vi "f_11_DvDtOff.vi"(0 "file path (IN)":path, 1 "Project #":string, 2 "Request #":string, 3 "TEST #":string, 5 "error in (no error)":errorcluster, 6 "VCE":dbl) -> (11 "Dv (V)":dbl, 13 "Dt (ns)":dbl, 14 "file path (OUT)":path, 15 "Dv/Dt (V/us)":dbl, 16 "DONE Dv/Dt OFF":bool, 19 "error out":errorcluster)   [LabVIEW 2020]
uses:
  GlobIndSw1.vi
  <vilib>/Waveform/WDTOps.llb/WDT Waveform Duration DBL.vi
  <vilib>/Waveform/WDTOps.llb/WDT Get Waveform Subset DBL.vi
  <vilib>/measure/mamon.llb/Trigger Detection for 1 Channel.vi
  <vilib>/Analysis/NI_AALBase.lvlib
  <vilib>/measure/NI_MAPro.lvlib
panel:
  in  "Decision ?":bool
  out "Dt (us)":dbl
  out "80% Vce":dbl
  out "50% Vce":dbl
  out "Cursor a : Channel 3":dbl
  out "Cursor b : Channel 3":dbl
  out "Waveform Graph":waveform(dbl)[](graph)
  out "OFF Region":waveform(dbl)[](graph) caption="DvDt off (V/us)"
  # "Dv/dt(off): from 50% to 80% of the peak voltage"
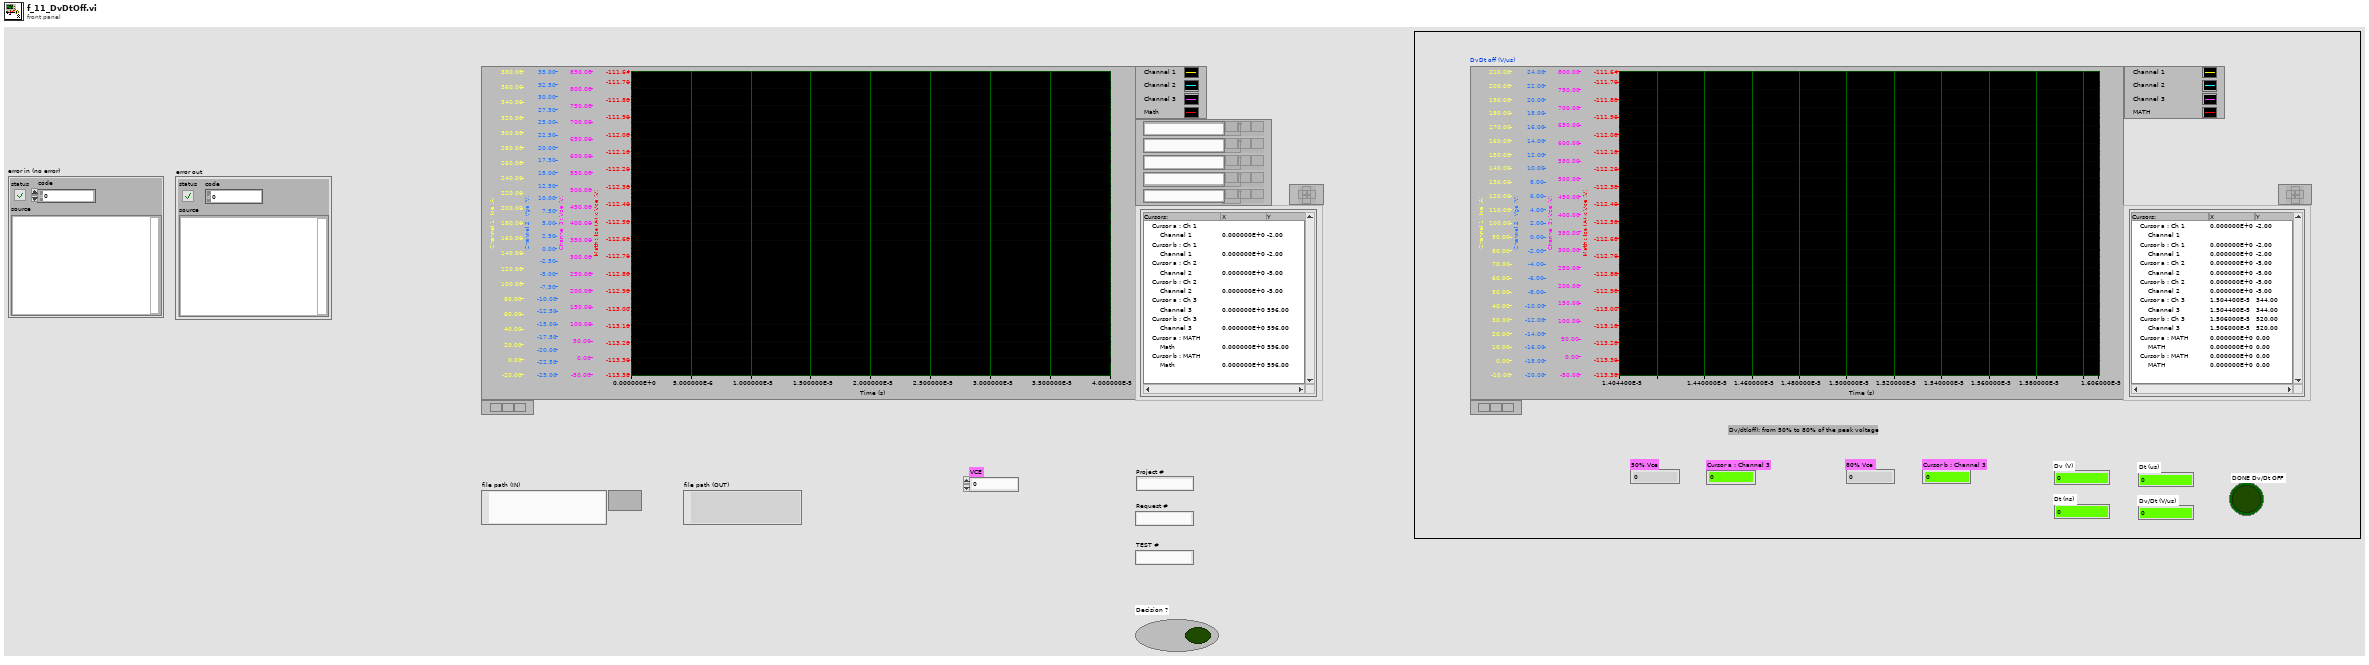
[diagram p1: front panel]
types:
  T1 = enum32{"Invalid", "Standard", "Closed", "Hidden", "Minimized", "Maximized"}
  T2 = typedef "imagedata.ctl" = cluster{"image type":i32, "image depth":i32, "image":u8[], "mask":u8[], "colors":u32[], "Rectangle":cluster{"left":i16, "top":i16, "right":i16, "bottom":i16}}
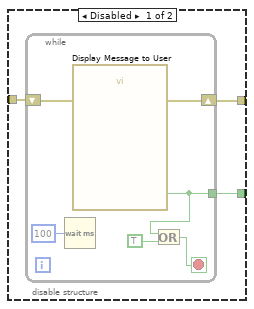
[diagram p2: hidden frame]
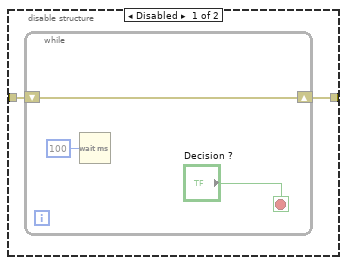
[diagram p7: hidden frame]
diagram:
  w2 = 0.0 ("Dv (V)")
  w3 = errorcluster {"status"=FALSE, "code"=0, "source"=""} ("error out")
  w1 = FALSE ("DONE Tdon")
  w4 = waveform(dbl)[] [] ("Waveform Graph")
  n1 = local write "error out"(w3) -> ()
  n2 = local write "error in (no error)"(w3) -> ()
  n3 = local write "DONE Dv/Dt OFF"(w1) -> ()
  n4 = local write "Waveform Graph"(w4) -> ()
  n5 = local write "OFF Region"(w4) -> ()
  n6 = local write "Decision ?"(w1) -> ()
  n7 = local write "Dv (V)"(w2) -> ()
  n8 = local write "Dt (ns)"(w2) -> ()
  n9 = local write "Dt (us)"(w2) -> ()
  n10 = local write "Dv/Dt (V/us)"(w2) -> ()
  n11 = local write "Cursor a : Channel 3"(w2) -> ()
  n12 = local write "Cursor b : Channel 3"(w2) -> ()
  n13 = flat-sequence {
    tunnel: ["error in (no error)"] -> w10
    tunnel: ["file path (IN)"] -> w9
    tunnel: [w21] -> w8
    tunnel: [w20] -> w7
    tunnel: w10 -> [w19]
    tunnel: w9 -> [w18]
    tunnel: [w279] -> w6
    tunnel: w8 -> [w278]
    tunnel: w7 -> [w277]
    tunnel: [w277] -> w5
    tunnel: w6 -> [w292]
    tunnel: w5 -> [w293]
    frame #0 {
      n14 = control-ref of="This VI"() -> (w15:refnum<vi>)
      n15 = invoke class="VI" method="FP.Open"(reference=w15, error in="error in (no error)", "Activate"=TRUE ("Activate?"), "State"=T1."Maximized") -> (error out=w16:errorcluster)  [unwired: 1 in, 4 out]
      n16 = property class="VI"(reference=w15, error in=w16, "Front Panel.Closeable"=TRUE ("Front Panel Window:Closeable")) -> ()  [unwired: 2 out]
    }
    frame #1 {
      n17 = while {
        shift-right: [w26] -> w21
        shift-left: w19 -> [w28]
        tunnel: [w23] -> w20
        tunnel: w18 -> [w22]
        stop <- w25 stop-if-true
        n18 = flat-sequence {
          tunnel: [w60] -> w47
          tunnel: w28 -> [w64]
          tunnel: [w64] -> w27
          tunnel: w22 -> [w60]
          tunnel: w47 -> [w155]
          tunnel: [w87] -> w46
          tunnel: [w77] -> w45
          tunnel: [w67] -> w44
          tunnel: w27 -> [w161]
          tunnel: w46 -> [w206]
          tunnel: [w216] -> w43
          tunnel: w45 -> [w225]
          tunnel: [w225] -> w42
          tunnel: [w213] -> w41
          tunnel: [w212] -> w40
          tunnel: [w199] -> w39
          tunnel: [w205] -> w38
          tunnel: w44 -> [w198]
          tunnel: w43 -> [w243]
          tunnel: [w244] -> w37
          tunnel: w42 -> [w247]
          tunnel: [w247] -> w36
          tunnel: w41 -> [w246]
          tunnel: [w246] -> w35
          tunnel: w40 -> [w245]
          tunnel: [w245] -> w34
          tunnel: w39 -> [w237]
          tunnel: [w237] -> w33
          tunnel: w38 -> [w238]
          tunnel: [w238] -> w32
          tunnel: w37 -> [w249]
          tunnel: w36 -> [w262]
          tunnel: [w262] -> w31
          tunnel: w35 -> [w256]
          tunnel: w34 -> [w257]
          tunnel: w33 -> [w255]
          tunnel: w32 -> [w254]
          tunnel: [w249] -> w30
          tunnel: w31 -> [w267]
          tunnel: w30 -> [w269]
          tunnel: [w268] -> w29
          tunnel: [w267] -> w23
          frame #0 {
            w62 = 0.0 ("Dv (V)")
            w63 = FALSE ("DONE Tdon")
            w61 = waveform(dbl)[] [] ("Waveform Graph")
            n19 = local write "DONE Dv/Dt OFF"(w63) -> ()
            n20 = local write "Dv (V)"(w62) -> ()
            n21 = local write "Dt (ns)"(w62) -> ()
            n22 = local write "Dt (us)"(w62) -> ()
            n23 = local write "Dv/Dt (V/us)"(w62) -> ()
            n24 = local write "Decision ?"(w63) -> ()
            n25 = local write "Cursor a : Channel 3"(w62) -> ()
            n26 = local write "Cursor b : Channel 3"(w62) -> ()
            n27 = Wait (ms)(milliseconds to wait=u32 400) -> ()  [unwired: 1 out]
            n28 = local write "Waveform Graph"(w61) -> ()
            n29 = local write "OFF Region"(w61) -> ()
          }
          frame #1 {
            w66 = 0.0 ("start samples/time")
            w136 = u16 1 items=["Samples", "Relative Time"] ("start/duration format")
            w147 = u16 1 items=["Samples", "Relative Time"] ("start/duration format")
            w148 = u16 1 items=["Samples", "Relative Time"] ("start/duration format")
            # "Channel 1"
            # "Channel 3"
            # "Channel 2"
            # "dt"
            # "Ch2"
            # "Ch1"
            n30 = call "3_ReadDatatoWaveform.vi"("error in (no error)"=w161, "file path (IN)"=w155) -> ("error out"=w70:errorcluster, "Waveform Graph"=→"Waveform Graph":waveform(dbl)[], "file path (OUT)"=w77:path, "dt"=w156:dbl, "Ch 2 Data"=w153:dbl[], "Ch 3 Data"=w157:dbl[], "Ch 1 Data"=w154:dbl[])  [unwired: 3 in]
            n31 = Wait (ms)(milliseconds to wait=u32 400) -> ()  [unwired: 1 out]
            n32 = call <vilib>:"Beep.vi"("use system alert? (T)"=FALSE, "duration (msec)"=u32 200, "frequency (Hz)"=u32 2000) -> ()  [unwired: 9 in]
            n33 = To Time Stamp(1:0.0 ("number")) -> (0:w158:timestamp)
            n34 = disable-structure shown="Enabled" {
              disable-tunnel: w158 -> [w181 _]
              disable-tunnel: w156 -> [w180 _]
              disable-tunnel: w154 -> [w179 _]
              disable-tunnel: [w178 _] -> w135
              frame Enabled {
                # "Channel 1"
                n35 = Bundle By Name("Y"=w179, "dt"=w180, "t0"=w181) -> (w178:waveform(dbl))  [unwired: 1 in]
              }
              frame Disabled {
              }
            }
            n36 = disable-structure shown="Enabled" {
              disable-tunnel: w158 -> [w185 _]
              disable-tunnel: w156 -> [w184 _]
              disable-tunnel: w153 -> [w183 _]
              disable-tunnel: [w182 _] -> w134
              frame Enabled {
                # "Channel 2"
                n37 = Bundle By Name("Y"=w183, "dt"=w184, "t0"=w185) -> (w182:waveform(dbl))  [unwired: 1 in]
              }
              frame Disabled {
              }
            }
            n38 = disable-structure shown="Enabled" {
              disable-tunnel: w158 -> [w189 _]
              disable-tunnel: w156 -> [w188 _]
              disable-tunnel: w157 -> [w187 _]
              disable-tunnel: [w186 _] -> w69
              frame Enabled {
                # "Channel 3"
                n39 = Bundle By Name("Y"=w187, "dt"=w188, "t0"=w189) -> (w186:waveform(dbl))  [unwired: 1 in]
              }
              frame Disabled {
              }
            }
            n40 = disable-structure shown="Enabled" {
              disable-tunnel: w69 -> [w174 _]
              disable-tunnel: w70 -> [w166 _]
              disable-tunnel: [w165 _] -> w71
              disable-tunnel: [w164 _] -> w67
              disable-tunnel: w66 -> [w163 _]
              frame Enabled {
                w168 = u16 1 items=["Samples", "Relative Time"] ("start/duration format")
                # "Channel 3 - Filtered"
                # "Median"
                n41 = global read "GlobIndSw1.vi" "Median Filter Rank"() -> (w162:i32)
                n42 = Unbundle By Name(w174) -> ("Y"=w177:dbl[], "dt"=w175:dbl)
                n43 = call <vilib>:"Median Filter.vi"("right rank"=w162, "left rank"=w162, "X"=w177) -> ("Filtered X"=w176:dbl[])  [unwired: 7 in, 1 out]
                n44 = Bundle By Name("Y"=w176, "dt"=w175) -> (w167:waveform(dbl))  [unwired: 1 in]
                n45 = call-poly <vilib>:"Waveform Duration.vi"("error in (no error)"=w166, "waveform in"=w167) -> ("error out"=w171:errorcluster, "duration"=w173:dbl, "waveform out"=w172:waveform(dbl))  [unwired: 7 in]
                n46 = Divide(x=w173, y=2.0) -> (x/y=w170:dbl)
                n47 = call-poly <vilib>:"Get Waveform Subset.vi"("start/duration format"=w168, "error in (no error)"=w171, "duration"=w170, "start samples/time"=w163, "waveform in"=w172) -> ("error out"=w165:errorcluster, "waveform out"=w164:waveform(dbl))  [unwired: 1 in, 2 out]
              }
              frame Disabled {
              }
            }
            n48 = call-poly <vilib>:"Waveform Duration.vi"("error in (no error)"=w70, "waveform in"=w69) -> ("error out"=w141:errorcluster, "duration"=w138:dbl, "waveform out"=w140:waveform(dbl))  [unwired: 7 in]
            n49 = call-poly <vilib>:"Waveform Duration.vi"("error in (no error)"=w70, "waveform in"=w134) -> ("error out"=w142:errorcluster, "duration"=w145:dbl, "waveform out"=w143:waveform(dbl))  [unwired: 7 in]
            n50 = call-poly <vilib>:"Waveform Duration.vi"("error in (no error)"=w70, "waveform in"=w135) -> ("error out"=w152:errorcluster, "duration"=w149:dbl, "waveform out"=w151:waveform(dbl))  [unwired: 7 in]
            n51 = Divide(x=w138, y=2.0) -> (x/y=w137:dbl)
            n52 = Divide(x=w145, y=2.0) -> (x/y=w146:dbl)
            n53 = Divide(x=w149, y=2.0) -> (x/y=w132:dbl)
            n54 = call-poly <vilib>:"Get Waveform Subset.vi"("start/duration format"=w136, "error in (no error)"=w141, "duration"=w137, "start samples/time"=w66, "waveform in"=w140) -> ("error out"=w68:errorcluster, "waveform out"=w73:waveform(dbl))  [unwired: 1 in, 2 out]
            n55 = call-poly <vilib>:"Get Waveform Subset.vi"("start/duration format"=w147, "error in (no error)"=w142, "duration"=w146, "start samples/time"=w66, "waveform in"=w143) -> ("error out"=w130:errorcluster, "waveform out"=w89:waveform(dbl))  [unwired: 1 in, 2 out]
            n56 = call-poly <vilib>:"Get Waveform Subset.vi"("start/duration format"=w148, "error in (no error)"=w152, "duration"=w132, "start samples/time"=w66, "waveform in"=w151) -> ("error out"=w131:errorcluster, "waveform out"=w88:waveform(dbl))  [unwired: 1 in, 2 out]
            n57 = Build Array(w88, w89, w73, waveform(dbl) {"t0"=timestamp(0 s since 1904-01-01), "dt"=1.0, "Y"=[]} ("element")) -> (→"OFF Region":waveform(dbl)[])
            n58 = Merge Errors(w131, w130, w68, w71) -> (w85:errorcluster)
            n59 = property on="OFF Region" class="WFGraph (strict)"(error in=w85) -> (error out=w84:errorcluster, "Width"=w83:u32)  [unwired: 1 in, 1 out]
            n60 = property on="OFF Region" class="WFGraph (strict)"(error in=w84, "Caption.Justify"=enum16{"Left", "Center", "Right"}."Left" ("Caption.Justification"), "Caption.Width"=w83, "Caption.FontBold"=TRUE ("Caption.Font:Bold"), "Caption.FontColor"=u32 16860 ("Caption.Font:Color"), "Caption.FontSize"=u32 24 ("Caption.Font:Size"), "Caption.Text"="DvDt off (V/us)") -> (error out=w79:errorcluster)  [unwired: 1 in, 1 out]
            n61 = property on="OFF Region" class="WFGraph (strict)"(error in=w79, "XScale.Offset"=w66) -> (error out=w113:errorcluster)  [unwired: 1 in, 1 out]
            n62 = property on="OFF Region" class="WFGraph (strict)"(error in=w113, "Active Cursor"=u32 0, "Cursor.Cursor X"=0.0 ("Cursor.Cursor Position:Cursor X"), "Cursor.Cursor Y"=0.0 ("Cursor.Cursor Position:Cursor Y"), "Cursor.Visible"=FALSE) -> (error out=w112:errorcluster)  [unwired: 1 in, 1 out]
            n63 = property on="OFF Region" class="WFGraph (strict)"(error in=w112, "Active Cursor"=u32 1, "Cursor.Cursor X"=0.0 ("Cursor.Cursor Position:Cursor X"), "Cursor.Cursor Y"=0.0 ("Cursor.Cursor Position:Cursor Y"), "Cursor.Visible"=FALSE) -> (error out=w111:errorcluster)  [unwired: 1 in, 1 out]
            n64 = property on="OFF Region" class="WFGraph (strict)"(error in=w111, "Active Cursor"=u32 2, "Cursor.Cursor X"=0.0 ("Cursor.Cursor Position:Cursor X"), "Cursor.Cursor Y"=0.0 ("Cursor.Cursor Position:Cursor Y"), "Cursor.Visible"=FALSE) -> (error out=w110:errorcluster)  [unwired: 1 in, 1 out]
            n65 = property on="OFF Region" class="WFGraph (strict)"(error in=w110, "Active Cursor"=u32 3, "Cursor.Cursor X"=0.0 ("Cursor.Cursor Position:Cursor X"), "Cursor.Cursor Y"=0.0 ("Cursor.Cursor Position:Cursor Y"), "Cursor.Visible"=FALSE) -> (error out=w93:errorcluster)  [unwired: 1 in, 1 out]
            n66 = property on="OFF Region" class="WFGraph (strict)"(error in=w93, "Active Cursor"=u32 4, "Cursor.Cursor X"=0.0 ("Cursor.Cursor Position:Cursor X"), "Cursor.Cursor Y"=0.0 ("Cursor.Cursor Position:Cursor Y"), "Cursor.Visible"=FALSE) -> (error out=w92:errorcluster)  [unwired: 1 in, 1 out]
            n67 = property on="OFF Region" class="WFGraph (strict)"(error in=w92, "Active Cursor"=u32 5, "Cursor.Cursor X"=0.0 ("Cursor.Cursor Position:Cursor X"), "Cursor.Cursor Y"=0.0 ("Cursor.Cursor Position:Cursor Y"), "Cursor.Visible"=FALSE) -> (error out=w91:errorcluster)  [unwired: 1 in, 1 out]
            n68 = property on="OFF Region" class="WFGraph (strict)"(error in=w91, "Active Cursor"=u32 6, "Cursor.Cursor X"=0.0 ("Cursor.Cursor Position:Cursor X"), "Cursor.Cursor Y"=0.0 ("Cursor.Cursor Position:Cursor Y"), "Cursor.Visible"=FALSE) -> (error out=w90:errorcluster)  [unwired: 1 in, 1 out]
            n69 = property on="OFF Region" class="WFGraph (strict)"(error in=w90, "Active Cursor"=u32 7, "Cursor.Cursor X"=0.0 ("Cursor.Cursor Position:Cursor X"), "Cursor.Cursor Y"=0.0 ("Cursor.Cursor Position:Cursor Y"), "Cursor.Visible"=FALSE) -> (error out=w87:errorcluster)  [unwired: 1 in, 1 out]
          }
          frame #2 {
            w203 = u16 1 items=["Falling Edge", "Rising Edge"] ("trigger slope")
            w204 = u16 1 items=["Index", "Time"] ("location mode")
            w210 = u16 1 items=["Falling Edge", "Rising Edge"] ("trigger slope")
            w211 = u16 1 items=["Index", "Time"] ("location mode")
            # "XPOS"
            # "YPOS"
            # "Cursor a : Channel 1"
            # "Cursor b : Channel 1"
            # "Cursor b : Channel 1"
            # "Cursor a : Channel 1"
            # "Cursor b : Channel 1"
            # "Cursor a : Channel 3"
            # "Cursor b : Channel 1"
            # "Cursor a : Channel 3"
            # "End Time 1st Cursor"
            # "End Time 2nd Cursor"
            # "1st PARAMETER : 50% Vce"
            # "Channel 1"
            # "2nd PARAMETER : 80% Vce"
            # "Channel 1"
            n70 = Wait (ms)(milliseconds to wait=u32 500) -> ()  [unwired: 1 out]
            n71 = call <vilib>:"Beep.vi"("use system alert? (T)"=FALSE, "duration (msec)"=u32 200, "frequency (Hz)"=u32 2000) -> ()  [unwired: 9 in]
            n72 = Divide(x=50.0, y=100.0) -> (x/y=w235:dbl)
            n73 = Multiply(x=w235, y="VCE") -> (x*y=w208:dbl)
            "50% Vce" <- w208
            n74 = Add(x=w208, y=0.2) -> (x+y=w196:dbl)
            n75 = Divide(x=w196, y=10.0) -> (x/y=w194:dbl)
            n76 = call-poly <vilib>:"Basic Level Trigger Detection.vi"("signal in"=w198, "level"=w196, "hysteresis"=w194, "location mode"=w211, "error in (no error)"=w206, "trigger slope"=w210) -> ("trigger location"=w205:dbl, "error out"=w207:errorcluster)  [unwired: 7 in, 1 out]
            n77 = property on="OFF Region" class="WFGraph (strict)"(error in=w207, "Active Cursor"=u32 4, "Cursor.Cursor X"=w205, "Cursor.Visible"=TRUE, "Cursor.Cursor Name Visible"=TRUE) -> (error out=w220:errorcluster)  [unwired: 1 in, 1 out]
            n78 = property on="OFF Region" class="WFGraph (strict)"(error in=w220, "Active Cursor"=u32 4) -> (error out=w201:errorcluster, "Cursor.Cursor Y"=w213:dbl)  [unwired: 1 in, 1 out]
            "Cursor a : Channel 3" <- w213
            n79 = Divide(x=80.0, y=100.0) -> (x/y=w232:dbl)
            n80 = Multiply(x=w232, y="VCE") -> (x*y=w197:dbl)
            "80% Vce" <- w197
            n81 = Add(x=w197, y=0.2) -> (x+y=w192:dbl)
            n82 = Divide(x=w192, y=10.0) -> (x/y=w191:dbl)
            n83 = call-poly <vilib>:"Basic Level Trigger Detection.vi"("signal in"=w198, "level"=w192, "hysteresis"=w191, "location mode"=w204, "error in (no error)"=w201, "trigger slope"=w203) -> ("trigger location"=w199:dbl, "error out"=w200:errorcluster)  [unwired: 7 in, 1 out]
            n84 = property on="OFF Region" class="WFGraph (strict)"(error in=w200, "Active Cursor"=u32 5, "Cursor.Cursor X"=w199, "Cursor.Visible"=TRUE, "Cursor.Cursor Name Visible"=TRUE) -> (error out=w217:errorcluster)  [unwired: 1 in, 1 out]
            n85 = property on="OFF Region" class="WFGraph (strict)"(error in=w217, "Active Cursor"=u32 5) -> (error out=w216:errorcluster, "Cursor.Cursor Y"=w212:dbl)  [unwired: 1 in, 1 out]
            "Cursor b : Channel 3" <- w212
          }
          frame #3 {
            # "2nd Cursor"
            # "1st Cursor"
            n86 = Subtract(x=w238, y=1e-06) -> (x-y=w240:dbl)
            n87 = Add(x=w237, y=1e-06) -> (x+y=w239:dbl)
            n88 = property on="OFF Region" class="WFGraph (strict)"(error in=w243, "XScale.Minimum"=w240, "XScale.Maximum"=w239) -> (error out=w244:errorcluster)  [unwired: 1 in, 1 out]
            n89 = Wait (ms)(milliseconds to wait=u32 300) -> ()  [unwired: 1 out]
          }
          frame #4 {
            # "us"
            # "ns"
            n90 = Subtract(x=w257, y=w256) -> (x-y=w253:dbl)
            n91 = Subtract(x=w255, y=w254) -> (x-y=w251:dbl)
            n92 = Absolute Value(x=w253) -> (abs(x)=w252:dbl)
            "Dv (V)" <- w252
            n93 = Absolute Value(x=w251) -> (abs(x)=w250:dbl)
            n94 = Multiply(x=w250, y=1000000000.0) -> (x*y=→"Dt (ns)":dbl)
            n95 = Multiply(x=w250, y=1000000.0) -> (x*y=w259:dbl)
            "Dt (us)" <- w259
            n96 = call <vilib>:"Beep.vi"("use system alert? (T)"=FALSE, "duration (msec)"=u32 200, "frequency (Hz)"=u32 2000) -> ()  [unwired: 9 in]
            n97 = Wait (ms)(milliseconds to wait=u32 300) -> ()  [unwired: 1 out]
            n98 = Divide(x=w252, y=w259) -> (x/y=→"Dv/Dt (V/us)":dbl)
          }
          frame #5 {
            n99 = disable-structure shown="Enabled" {
              disable-tunnel: w269 -> [w271 w275]
              disable-tunnel: [w270 w275] -> w268
              frame Disabled {
                n100 = while {
                  shift-right: [w272] -> w270
                  shift-left: w271 -> [w272]
                  stop <- "Decision ?" stop-if-true
                  n101 = Wait (ms)(milliseconds to wait=u32 100) -> ()  [unwired: 1 out]
                }
              }
              frame Enabled {
              }
            }
          }
        }
        n102 = disable-structure shown="Enabled" {
          disable-tunnel: w29 -> [w50 w58]
          disable-tunnel: [w49 w58] -> w26
          disable-tunnel: [w48 TRUE ("NO")] -> w25
          frame Disabled {
            n103 = while {
              tunnel: [w52] -> w48
              shift-right: [w55] -> w49
              shift-left: w50 -> [w56]
              stop <- w54 stop-if-true
              n104 = Wait (ms)(milliseconds to wait=u32 100) -> ()  [unwired: 1 out]
              n105 = call "Display Message to User"("error in (no error)"=w56) -> ("error out"=w55:errorcluster, "NO"=w52:bool)  [unwired: 9 in]
              n106 = Or(x=w52, y=TRUE) -> (x .or. y?=w54:bool)
            }
          }
          frame Enabled {
          }
        }
        n107 = Wait (ms)(milliseconds to wait=u32 100) -> ()  [unwired: 1 out]
      }
    }
    frame #2 {
      w282 = "_"
      n108 = Wait (ms)(milliseconds to wait=u32 300) -> ()  [unwired: 1 out]
      n109 = invoke on="OFF Region" class="WFGraph (strict)" method="Get Image"(error in=w278) -> (error out=w285:errorcluster, "image data"=w288:T2)  [unwired: 5 in, 4 out]
      n110 = Concatenate Strings("C:\\Inductive_Switching_Project\\IndSw_Image\\" ("string"), "Project #", w282, "Request #", w282, "TEST #", w282, "DvDtoff" ("string"), ".png" ("string")) -> (w289:string)
      n111 = String To Path(string=w289) -> (path=w287:path)
      n112 = call <vilib>:"Write PNG File.vi"("error in (no error)"=w285, "image data"=w288, "path to PNG file"=w287) -> ("error out"=w279:errorcluster)  [unwired: 7 in, 1 out]
      "DONE Dv/Dt OFF" <- TRUE ("DONE Di/Dt ON")
    }
    frame #3 {
      n113 = disable-structure shown="Enabled" {
        disable-tunnel: w292 -> [w294 _]
        frame Enabled {
          n114 = control-ref of="This VI"() -> (w295:refnum<vi>)
          n115 = invoke class="VI" method="FP.Close"(reference=w295, error in=w294) -> ()  [unwired: 1 in, 3 out]
        }
        frame Disabled {
        }
      }
      "error out" <- w292
      "file path (OUT)" <- w293
    }
  }
